vi "HAL camera info.vi"(2 "error in":errorcluster) -> (0 "error out":errorcluster, 1 "Andor Camera Properties":T2)   [LabVIEW 2011]
uses:
  HAL camera properties.ctl
  Cascade-specific globals.vi
panel:
  out "Camera Specific Versions":T1
  out "Camera Handle":u32
  # "Camera:  Roper Cascade"
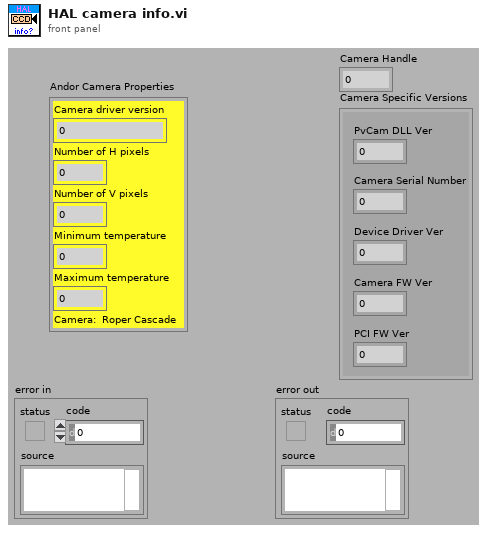
[diagram p1: front panel]
types:
  T1 = cluster{"PvCam DLL Ver":u32, "Camera Serial Number ":u32, "Device Driver Ver":u32, "Camera FW Ver":u32, "PCI FW Ver":u32}
  T2 = typedef "HAL camera properties.ctl" = cluster{"Camera driver version":u64, "Number of H pixels":i32, "Number of V pixels":i32, "Minimum temperature":i32, "Maximum temperature":i32}
  T3 = cluster{"Camera Handle":u32, "Pulser Handle":u32, "File Handle":u32, "Display Handle":u32, "Image Handle":u32}
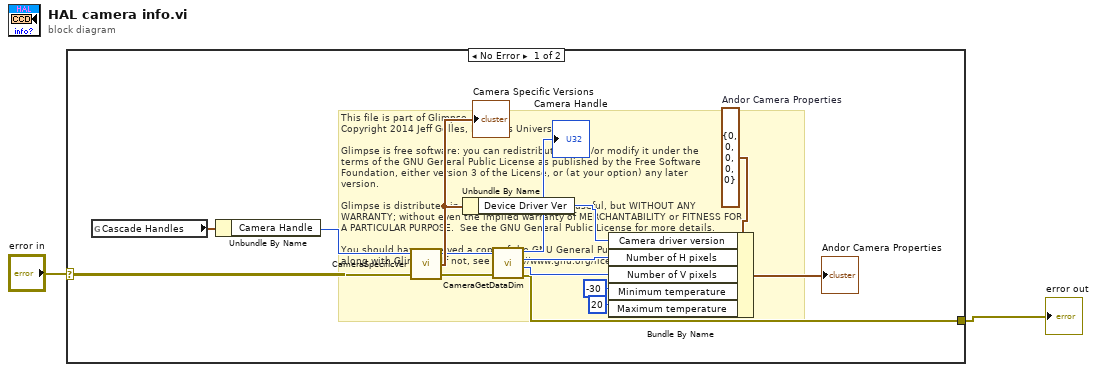
[diagram p0: block diagram]
diagram:
  # "This file is part of Glimpse. \nCopyright 2014 Jeff Gelles, Brandeis University.    \n\nGlimpse is free software: you can redistribute it and/or modify it under the \nterms of the GNU General Public License as published by the Free Software \nFoundation, either version 3 of the License, or (at your option) any later \nversion.\n\nGlimpse is distributed in the hope that it will be useful, but WITHOUT ANY \nWARRANTY; without even the implied warranty of MERCHANTABILITY or FITNESS FOR \nA PARTICULAR PURPOSE.  See the GNU General Public License for more details.\n\nYou should have received a copy of the GNU General Public License\nalong with Glimpse.  If not, see <http://www.gnu.org/licenses/>."
  n1 = case shown="No Error" "error in" {
    selector: "error in" -> [w16 w18]
    tunnel: [w7 w18] -> w1
    frame No Error {
      w14 = T2 {"Camera driver version"=0, "Number of H pixels"=0, "Number of V pixels"=0, "Minimum temperature"=0, "Maximum temperature"=0}  # Andor Camera Properties
      n2 = global read "Cascade-specific globals.vi" "Cascade Handles"() -> (w6:T3)
      n3 = Unbundle By Name(w6) -> ("Camera Handle"=w5:u32)
      n4 = call <userlib>:"CameraSpecificVer.vi"("error in (no error)"=w16, "Camera Handle"=w5) -> ("error out"=w15:errorcluster, "Camera Specific Versions"=w17:T1, "Camera Handle"=w4:u32)  [unwired: 1 out]
      "Camera Specific Versions" <- w17
      n5 = Unbundle By Name(w17) -> ("Device Driver Ver"=w12:u32)
      n6 = call <userlib>:"CameraGetDataDim.vi"("Camera Handle"=w4, "error in"=w15) -> ("Camera Handle"=→"Camera Handle":u32, "Xdim"=w11:u32, "Ydim"=w10:u32, "error out"=w7:errorcluster)
      n7 = Bundle By Name(cluster=w14, "Camera driver version"=w12, "Number of H pixels"=w11, "Number of V pixels"=w10, "Minimum temperature"=-30, "Maximum temperature"=20) -> (→"Andor Camera Properties":T2)
    }
    frame Error {
    }
  }
  "error out" <- w1
